vi "fill corners.vi"(11 "intensity values":dbl[][](array[numeric])) -> (3 "Array":dbl[][](array[numeric]))   [LabVIEW 2016]
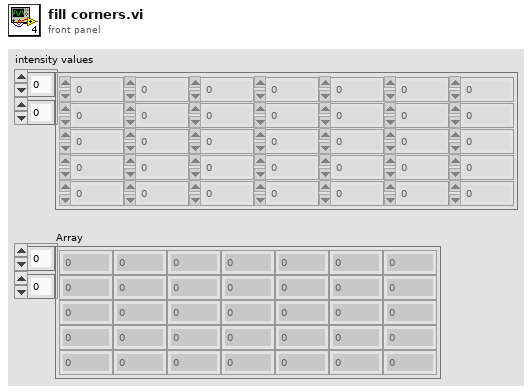
[diagram p1: front panel]
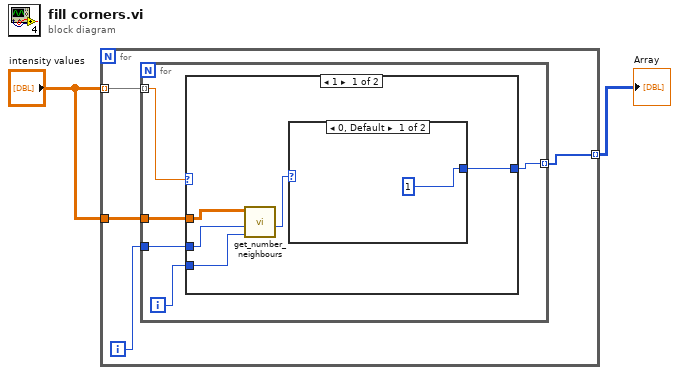
[diagram p0: block diagram]
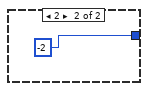
[diagram p2: hidden frame]
diagram:
  n1 = for {
    tunnel: "intensity values" -> [w6] mode=indexing
    tunnel: "intensity values" -> [w4]
    tunnel: [w3] -> w1 mode=indexing
    i -> [w5]
    n2 = for {
      tunnel: w6 -> [w11] mode=indexing
      tunnel: w5 -> [w10]
      tunnel: w4 -> [w8]
      tunnel: [w7] -> w3 mode=indexing
      i -> [w9]
      n3 = case shown="1" w11 {
        selector: w11 -> [_ w19]
        tunnel: w10 -> [w15 _]
        tunnel: w9 -> [w14 _]
        tunnel: w8 -> [w16 _]
        tunnel: [w12 w19] -> w7
        frame 1 {
          n4 = call "get_number_neighbours.vi"("index2"=w14, "index1"=w15, "Array"=w16) -> ("Numeric"=w13:i32)  [unwired: 8 in]
          n5 = case shown="0, Default" w13 {
            tunnel: [1 -2] -> w12
            frame 0, Default {
            }
            frame 2 {
            }
          }
        }
        frame Default {
        }
      }
    }
  }
  "Array" <- w1
